vi "Digital_Voltmeter (2024 Version).vi"() -> ()   [LabVIEW 2024]
panel:
  in  "stop":bool
  out "Voltage Over Time":dbl(graph)
  out "Voltage Reading (V)":dbl
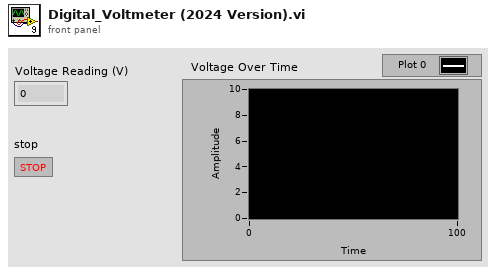
[diagram p1: front panel]
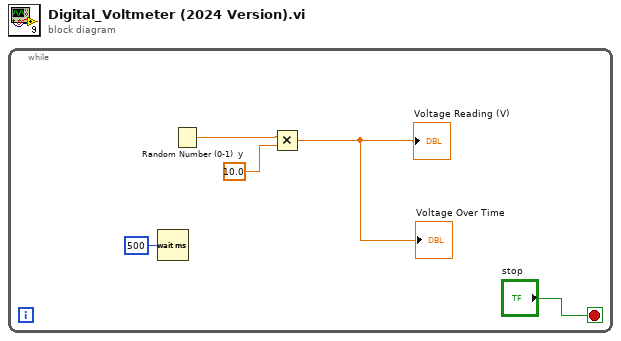
[diagram p0: block diagram]
diagram:
  n1 = while {
    stop <- "stop" stop-if-true
    w4 = 10.0  # y
    n2 = Wait (ms)(milliseconds to wait=u32 500) -> ()  [unwired: 1 out]
    n3 = Random Number (0-1)() -> (number: 0 to 1=w5:dbl)
    n4 = Multiply(x=w5, y=w4) -> (x*y=→"Voltage Reading (V)" →"Voltage Over Time":dbl)
  }
